vi "GetEnumValue.vi"(8 "error in (no error)":errorcluster caption="错误输入（无错误）", 10 "strKey":string, 11 "handle":u64) -> (0 "error out":errorcluster caption="错误输出", 1 "pEnumValue out":T1, 2 "function return":i32 format="%x", 3 "handle out":u64)   [LabVIEW 2013, in "MvCameraControl.lvlib"]
doc: "MV_LV_API int __stdcall GetEnumValue( void* handle, const char* strValue, MVCC_ENUMVALUE *pEnumValue);"
uses:
  MvCameraControl.lvlib
  MvCameraPatch.dll
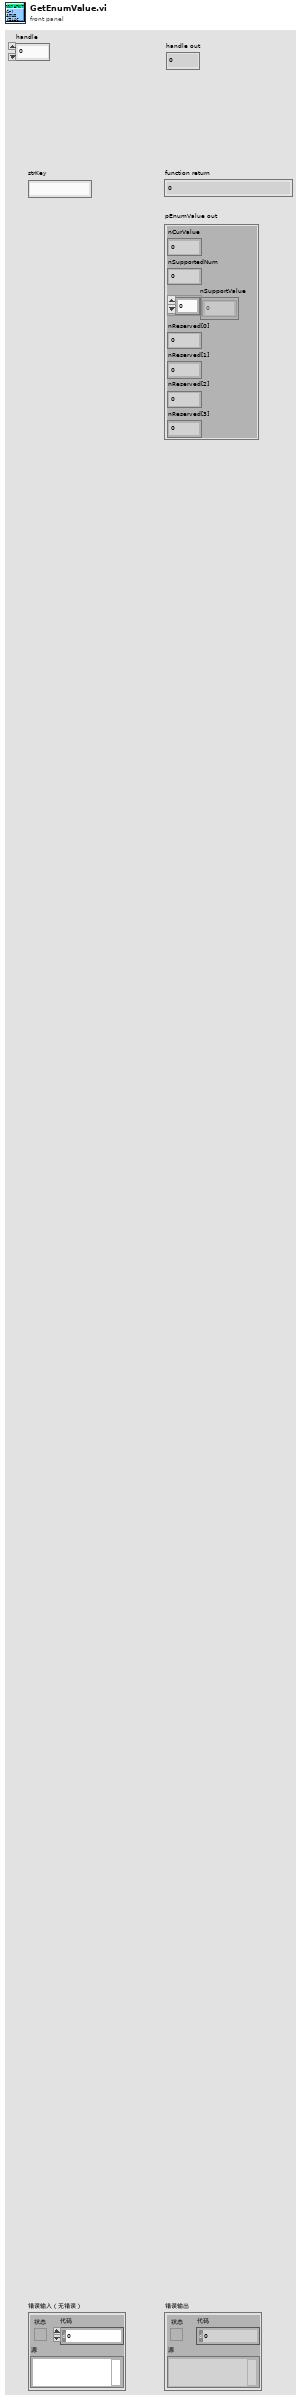
[diagram p1: front panel]
types:
  T1 = cluster{"nCurValue":u32, "nSupportedNum":u32, "nSupportValue":u32[], "nReserved[0]":u32, "nReserved[1]":u32, "nReserved[2]":u32, "nReserved[3]":u32}
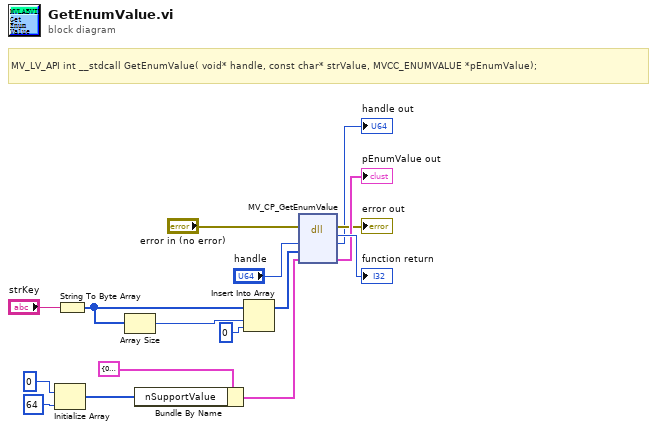
[diagram p0: block diagram]
diagram:
  # "MV_LV_API int __stdcall GetEnumValue( void* handle, const char* strValue, MVCC_ENUMVALUE *pEnumValue);"
  n1 = Initialize Array(u32 0 ("element"), 64 ("dimension size")) -> (w2:u32[])
  n2 = String To Byte Array(string="strKey") -> (unsigned byte array=w12:u8[])
  n3 = Array Size(array=w12) -> (size(s)=w11:i32)
  n4 = Bundle By Name(cluster=T1 {"nCurValue"=0, "nSupportedNum"=0, "nSupportValue"=[], "nReserved[0]"=0, "nReserved[1]"=0, "nReserved[2]"=0, "nReserved[3]"=0} ("pEnumValue out"), "nSupportValue"=w2) -> (w1:T1)
  n5 = Insert Into Array(array=w12, index=w11, new element=u8 0 ("新元素/子数组")) -> (w8:u8[])
  n6 = dll-call lib="MvCameraPatch.dll" fn="MV_CP_GetEnumValue"(error in="error in (no error)", "handle"="handle", "strKey"=w8, "pEnumValue"=w1) -> (error out=→"error out":errorcluster, "返回类型"=→"function return":i32, "handle"=→"handle out":u64, "pEnumValue"=→"pEnumValue out":T1)  [unwired: 3 in, 1 out]
